vi "Deserialize an Object with Type Information (Inline).vi"() -> ()   [LabVIEW 2017]
doc: "Demonstrates the JSONtext Object Serializer by deserializing a LabVIEW Object from a JSON Object with type information."
uses:
  Generic Object Serializer/Generic Object Serializer.lvclass
  C:/Program Files (x86)/National Instruments/LabVIEW 2017/vi.lib/JDP Science/JSONtext/LVClass Serializer/JSONtext LVClass Serializer.lvclass
  Account/Account.lvclass
  Generic Object Serializer/Type Name Handling.ctl
  Generic Object Serializer/Generic Object Serializer.lvclass/Generic Object Serializer.ctl
  c1b321db-ba44-4e46-b14b-83a8d0196014.vi
  Generic Object Serializer/Write Type Name Handling.vi
  <vilib>/JDP Science/JSONtext/JSON text to Variant.vi
panel:
  out "Summary":string
  out "error out":errorcluster
  in  "<JSON>":string="{\n  \"$type\":\"Account.lvclass\",\n  \"Email\":\"john.doe@example.com\",\n  \"Active\":true,\n  \"CreatedDate\":\"2021-04-03T06:30:00.000Z\",\n  \"Roles\":[\"User\",\"Admin\"]\n}"
  # "Overview\nDemonstrates the JSONtext Object Serializer by deserializing a LabVIEW Object from a JSON Object with type information.\n\nInstructions\nRun the VI"
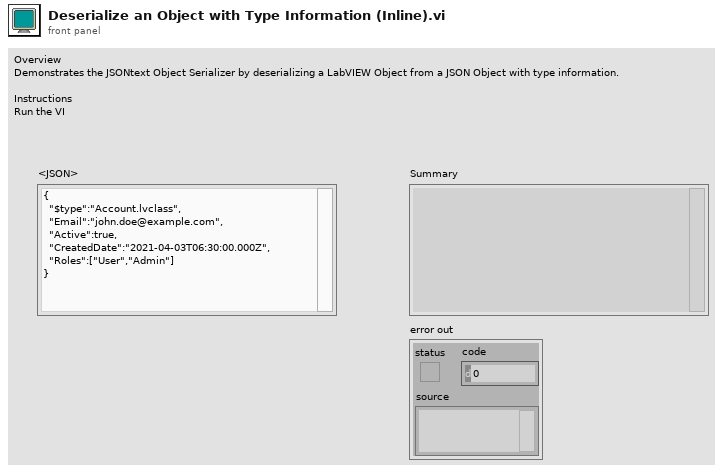
[diagram p1: front panel]
types:
  T1 = typedef "Generic Object Serializer.lvclass/Type Name Handling.ctl" = enum16{"None", "Inline"}
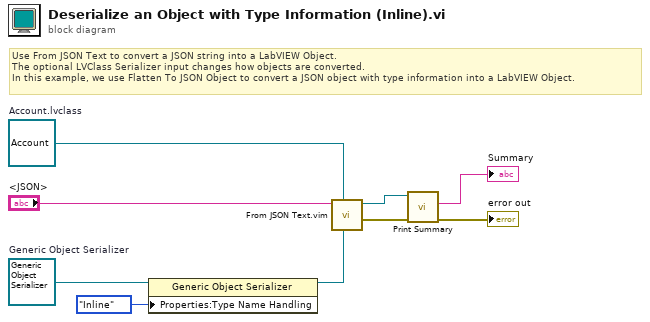
[diagram p0: block diagram]
diagram:
  w6 = refnum<class "Account.lvclass"> refnum  # Account.lvclass
  w8 = refnum<class "Generic Object Serializer.lvclass"> refnum  # Generic Object Serializer
  # "Use From JSON Text to convert a JSON string into a LabVIEW Object.\nThe optional LVClass Serializer input changes how objects are converted.\nIn this example, we use Flatten To JSON Object to convert a JSON object with type information into a LabVIEW Object."
  n1 = property class="Generic Object Serializer"(reference=w8, "Properties:Type Name Handling"=Type_Name_Handling."Inline" ("Type Name Handling")) -> (reference out=w2:refnum<class "Generic Object Serializer.lvclass">)  [unwired: 1 in, 1 out]
  n2 = call "From JSON Text.vim"("LVClass Serializer"=w2, "Data Type and Default Value"=w6, "JSON"="<JSON>") -> ("error out"=w9:errorcluster, "Data out"=w4:refnum<class "Account.lvclass">)  [unwired: 7 in]
  n3 = call "Print Summary.vi"("error in (no error)"=w9, "Account in"=w4) -> ("error out"=→"error out":errorcluster, "Summary"=→"Summary":string)  [unwired: 7 in, 1 out]
